vi "receiveHealthAndStatus.vi"(8 "error in (no error)":errorcluster, 10 "Address":u32, 11 "RTHealthAndStatus in":refnum<class "RTHealthAndStatus.lvclass">) -> (0 "error out":errorcluster, 2 "Data":u32, 3 "RTHealthAndStatus out":refnum<class "RTHealthAndStatus.lvclass">)   [LabVIEW 2016, in "RTHealthAndStatus.lvlib" / "RTHealthAndStatus.lvclass"]
uses:
  RTHealthAndStatus.lvclass
  RTHealthAndStatus.lvclass/RTHealthAndStatus.ctl
  Common_RT_FPGA/IReadU32FIFO/IReadU32FIFO.lvclass
  Common_RT_FPGA/IWriteU64FIFO/IWriteU64FIFO.lvclass
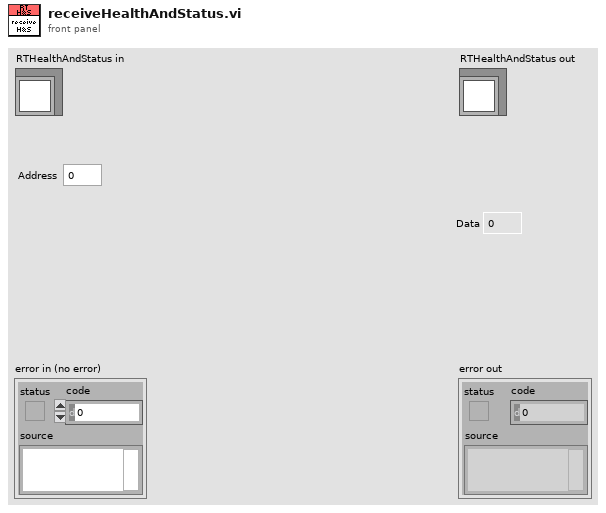
[diagram p1: front panel]
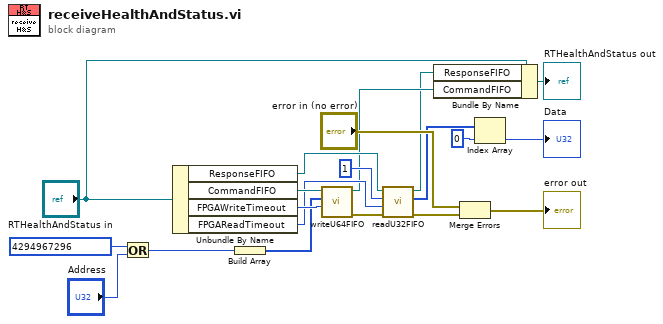
[diagram p0: block diagram]
diagram:
  n1 = Or(x=u64 4294967296, y="Address") -> (x .or. y?=w16:u64)
  n2 = Unbundle By Name("RTHealthAndStatus in") -> ("ResponseFIFO"=w6:refnum<class "IReadU32FIFO.lvclass">, "CommandFIFO"=w13:refnum<class "IWriteU64FIFO.lvclass">, "FPGAWriteTimeout"=w14:i32, "FPGAReadTimeout"=w10:i32)
  n3 = Build Array(w16) -> (w12:u64[])
  n4 = call-dynamic "writeU64FIFO.vi"("Timeout"=w14, "Data"=w12, "IWriteU64FIFO in"=w13) -> ("error out"=w11:errorcluster, "IWriteU64FIFO out"=w3:refnum<class "IWriteU64FIFO.lvclass">)  [unwired: 6 in, 1 out]
  n5 = call-dynamic "readU32FIFO.vi"("error in (no error)"=w11, "Timeout"=w10, "NumberOfElements"=u32 1 ("Number of Elements"), "IReadU32FIFO in"=w6) -> ("error out"=w7:errorcluster, "Data"=w8:u32[], "IReadU32FIFO out"=w2:refnum<class "IReadU32FIFO.lvclass">)  [unwired: 4 in, 1 out]
  n6 = Bundle By Name(cluster="RTHealthAndStatus in", "ResponseFIFO"=w2, "CommandFIFO"=w3) -> (→"RTHealthAndStatus out":refnum<class "RTHealthAndStatus.lvclass">)
  n7 = Merge Errors("error in (no error)", w7) -> (→"error out":errorcluster)
  n8 = Index Array(array=w8, index=0) -> (element=→"Data":u32)
